vi "read full data dictionary.vi"(8 "error in":errorcluster, 11 "data dictionary in":refnum<class "data bus dictionary.lvclass">) -> (0 "error out":errorcluster, 2 "elements":cluster{"name":string, "dictionary lookup":T1}[](array[cluster]), 3 "data dictionary out":refnum<class "data bus dictionary.lvclass">)   [LabVIEW 2013, in "data bus dictionary.lvclass"]
doc: "Reads the entire data dictionary and returns it as a sorted set of tag names, organized by data type. This is very inefficient, duplicating the entire tag list and performing a sorting algorithm on this list."
uses:
  data bus dictionary.lvclass
  dictionary lookup value.ctl
  tag/Data Type.ctl
  data bus dictionary.lvclass/data bus dictionary.ctl
  tag/data bus tag description.lvclass
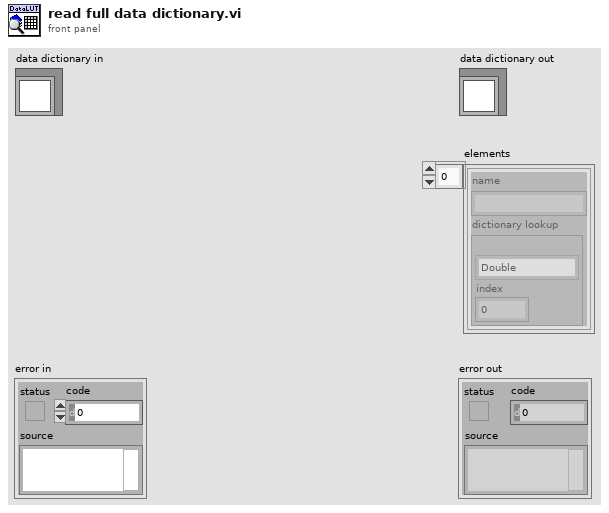
[diagram p1: front panel]
types:
  T1 = typedef "data bus dictionary.lvclass/dictionary lookup value.ctl" = cluster{"data type":T2, "index":i32}
  T2 = typedef "data bus tag description.lvclass/Data Type.ctl" = enum16{"Double", "I64", "Boolean", "Array of Double", "Array of I64", "Variant"}
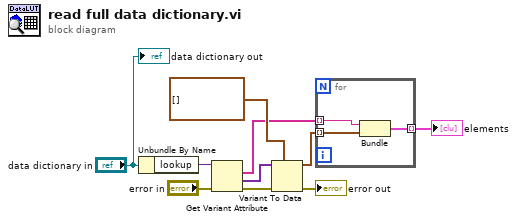
[diagram p0: block diagram]
diagram:
  n1 = Unbundle By Name("data dictionary in") -> ("lookup"=w9:variant)
  n2 = Get Variant Attribute(Variant=w9, error in="error in") -> (names=w3:string[], values=w7:variant[], error out=w6:errorcluster)  [unwired: 2 in, 1 out]
  n3 = Variant To Data(error in=w6, type=T1[] [] ("elements"), Variant=w7) -> (data=w2:T1[], error out=→"error out":errorcluster)
  n4 = for {
    tunnel: w3 -> [w13] mode=indexing
    tunnel: w2 -> [w12] mode=indexing
    tunnel: [w11] -> w1 mode=indexing
    n5 = Bundle(w13, "dictionary lookup"=w12) -> (w11:cluster{string, "dictionary lookup":T1})  [unwired: 1 in]
  }
  "elements" <- w1
  "data dictionary out" <- "data dictionary in"
